vi "SngJntArmSim_WouldHitUpperLimit.vi"(10 "Angle_Rad":dbl=1.0, 11 "SingleJointArmSim":T1 {"GearBox"."Jr_KgM2" format="%13.5p"; "GearBox"."L_H" format="%13.5p"; "GearBox"."Kt_NMPerAmp" format="%13.5p"; "GearBox"."KvINV_RadPerSecPerVolt" format="%13.5p"; "GearBox"."R_Ohms" format="%13.5p"; "GearBox"."FreeSpeed_RadPerSec" format="%13.5p"; "GearBox"."FreeCurrent_Amps" format="%13.5p"; "GearBox"."StallCurrent_Amps" format="%13.5p"; "GearBox"."StallTorque_NM" format="%13.5p"; "GearBox"."nominalVoltage_Volts" format="%13.5p"}) -> (3 "Would Hit HIgh LImit":bool)   [LabVIEW 2019, in "Trajectory_Library.lvlib"]
doc: "Returns whether the arm has hit the upper limit.\n \nInputs:\n - SingleJointArmSim -- updated system data cluster\n - currentAngleRads -- The current arm height.\n\nOutputs:\n - WouldHitHighLimit -- Whether the arm would hit the upper limit."
uses:
  Trajectory_Library.lvlib
  SINGLE_JOINT_ARM_SIM.ctl
  LINEAR_SYSTEM_SIM.ctl
  LINEAR_SYSTEM.ctl
  <vilib>/Analysis/Matrix/Datatypes/RealMatrix.ctl
  DCMOTOR.CTL
  <vilib>/Analysis/Matrix/NI_Matrix.lvlib
panel:
  # "<States, 1>"
  # "<Outputs, 1>"
  # "<Inputs, 1>"
  # "<Outputs, 1>"
  # "<States,States>"
  # "<States,Inputs>"
  # "<Outputs,States>"
  # "<Outputs,Inputs>"
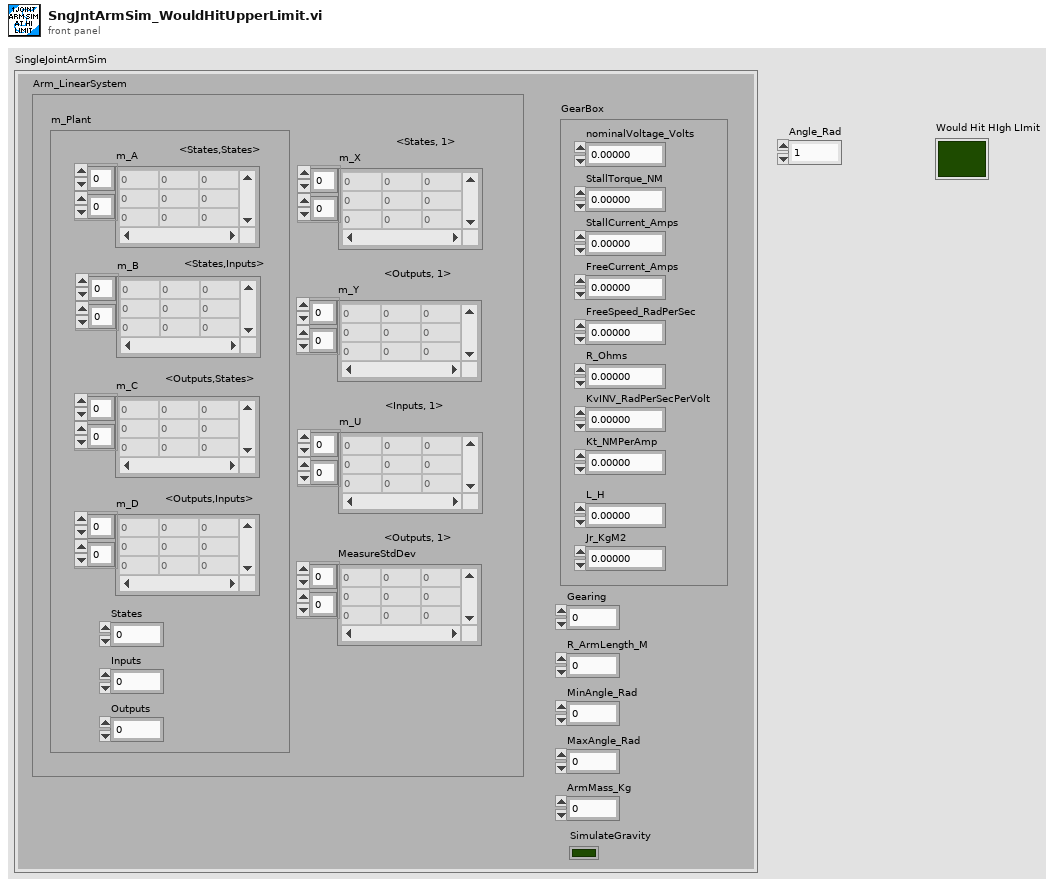
[diagram p1: front panel]
types:
  T1 = typedef "Trajectory_Library.lvlib/SINGLE_JOINT_ARM_SIM.ctl" = cluster{"Arm_LinearSystem":T2, "GearBox":T5, "Gearing":dbl, "R_ArmLength_M":dbl, "MinAngle_Rad":dbl, "MaxAngle_Rad":dbl, "ArmMass_Kg":dbl, "SimulateGravity":bool}
  T2 = typedef "Trajectory_Library.lvlib/LINEAR_SYSTEM_SIM.ctl" = cluster{"m_Plant":T3, "m_X":T4, "m_Y":T4, "m_U":T4, "MeasureStdDev":T4}
  T3 = typedef "Trajectory_Library.lvlib/LINEAR_SYSTEM.ctl" = cluster{"m_A":T4, "m_B":T4, "m_C":T4, "m_D":T4, "States":i32, "Inputs":i32, "Outputs":i32}
  T4 = typedef "NI_Matrix.lvlib/RealMatrix.ctl" = dbl[][]
  T5 = typedef "Trajectory_Library.lvlib/DCMOTOR.CTL" = cluster{"nominalVoltage_Volts":dbl, "StallTorque_NM":dbl, "StallCurrent_Amps":dbl, "FreeCurrent_Amps":dbl, "FreeSpeed_RadPerSec":dbl, "R_Ohms":dbl, "KvINV_RadPerSecPerVolt":dbl, "Kt_NMPerAmp":dbl, "L_H":dbl, "Jr_KgM2":dbl}
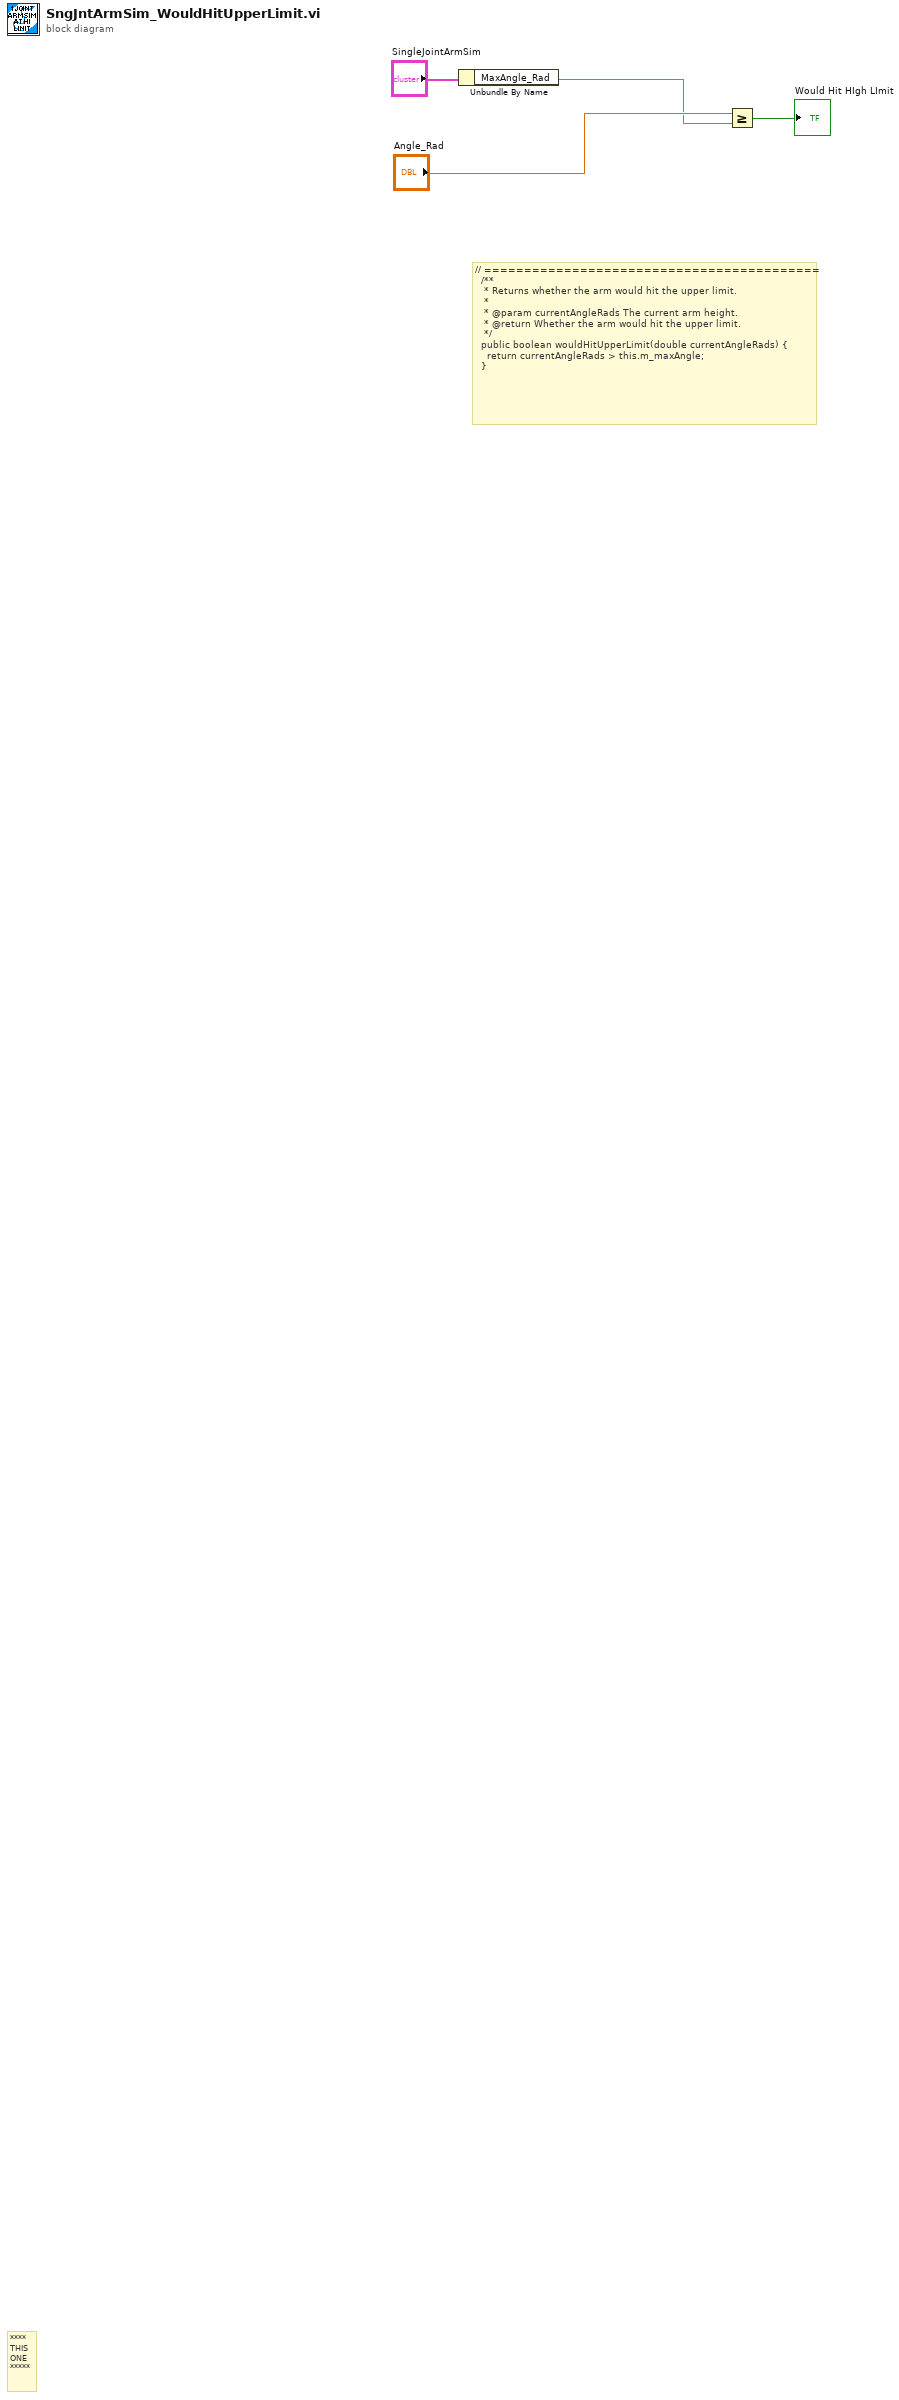
[diagram p0: block diagram]
diagram:
  # "// ==========================================\n  /**\n   * Returns whether the arm would hit the upper limit.\n   *\n   * @param currentAngleRads The current arm height.\n   * @return Whether the arm would hit the upper limit.\n   */\n  public boolean wouldHitUpperLimit(double currentAngleRads) {\n    return currentAngleRads > this.m_maxAngle;\n  }"
  # "****\nTHIS\nONE\n*****"
  n1 = Unbundle By Name("SingleJointArmSim") -> ("MaxAngle_Rad"=w1:dbl)
  n2 = Greater Or Equal?(x="Angle_Rad", y=w1) -> (x >= y?=→"Would Hit HIgh LImit":bool)
